vi "Write Application Settings.vi"(8 "error in":errorcluster, 10 "Application Settings":T4={"Storage Settings"={"Primary Path"=path "", "Backup Storage?"=FALSE, "Backup Path"=path "", "Component Name Prefix"="", "Image Format"=enum."<Select>"}, "PLC Settings"={"Port"="", "BaudRate"=9600, "Wakeup Signal Address "=0, "Acquisiton Address"=0, "Acknowledgement Address"=0, "Sleep Address"=0}, "Total Images"=0}, 11 "Controller in":refnum<class "Controller.lvclass">) -> (0 "error out":errorcluster, 3 "Controller out":refnum<class "Controller.lvclass">)   [LabVIEW 2021, in "Controller.lvlib" / "Controller.lvclass"]
uses:
  Controller.lvclass
  Typedefs/Image Formats.ctl
  Typedefs/Storage Settings.ctl
  Typedefs/PLC Settings.ctl
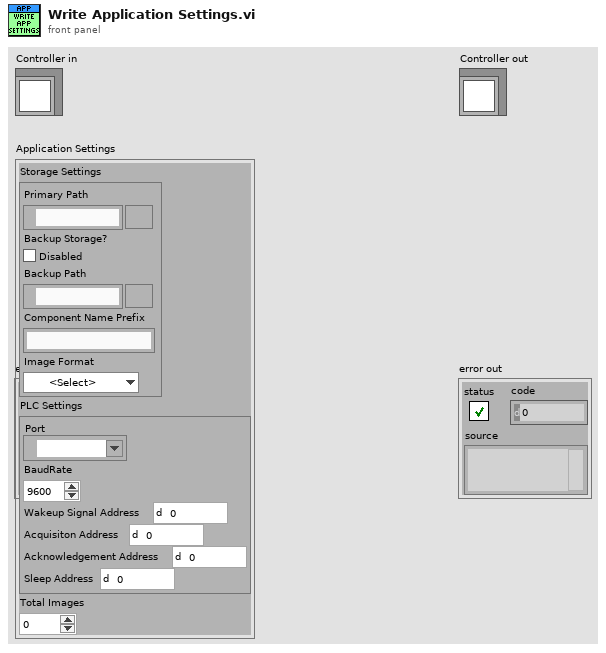
[diagram p1: front panel]
types:
  T1 = typedef "Storage Settings.ctl" = cluster{"Primary Path":path, "Backup Storage?":bool, "Backup Path":path, "Component Name Prefix":string, "Image Format":T2}
  T2 = typedef "Image Formats.ctl" = enum16{"<Select>", "TIFF", "RAW"}
  T3 = typedef "PLC Settings.ctl" = cluster{"Port":refnum<visa-resource-name>, "BaudRate":u32, "Wakeup Signal Address ":u16, "Acquisiton Address":u16, "Acknowledgement Address":u16, "Sleep Address":u16}
  T4 = cluster{"Storage Settings":T1, "PLC Settings":T3, "Total Images":u32}
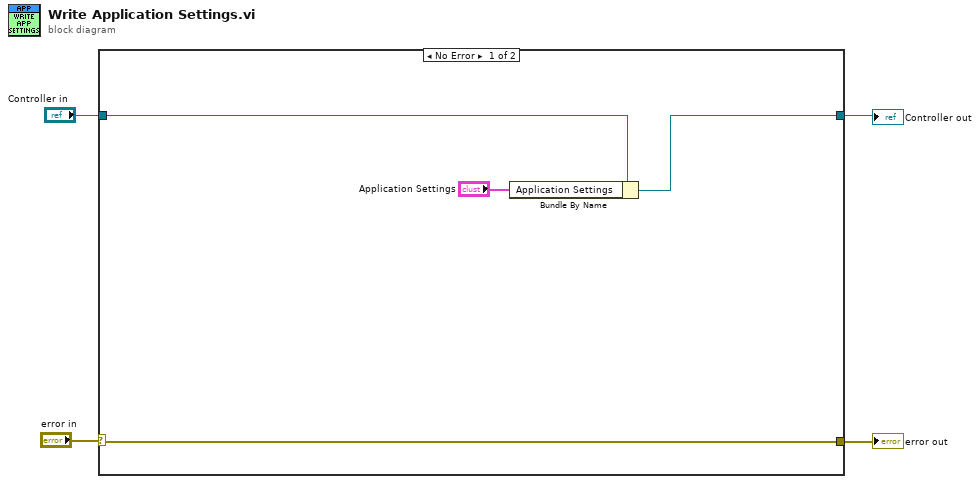
[diagram p0: block diagram]
diagram:
  n1 = case shown="No Error" "error in" {
    selector: "error in" -> [w8 w9]
    tunnel: [w8 w9] -> w4
    tunnel: [w6 w10] -> w3
    tunnel: "Controller in" -> [w7 w10]
    frame No Error {
      n2 = Bundle By Name(cluster=w7, "Application Settings"="Application Settings") -> (w6:refnum<class "Controller.lvclass">)
    }
    frame Error {
    }
  }
  "error out" <- w4
  "Controller out" <- w3
